vi "motionMagicConfig.vi"() -> ()   [LabVIEW 2018]
uses:
  conversionTypeEnum.ctl
  Constants.vi
panel:
  out "Max Velocity (Inches)":dbl=3.9081455805892547
  in  "D":dbl
  in  "I":dbl
  in  "P":dbl=3.0
  in  "Acceleration":i32=6000
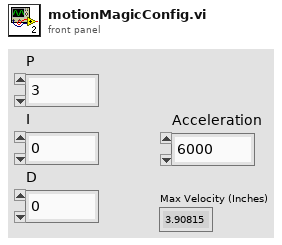
[diagram p1: front panel]
types:
  T1 = typedef "conversionTypeEnum.ctl" = enum16{"Sensor Units -> Inches", "Inches -> Sensor Units"}
  T2 = typedef "WPI_MotorControlDeviceRef.ctl" = cluster{"DeviceStatus":errorcluster, "Type":T3, "PWM":cluster{"PWM Channel":T4, "DeadBand":T5}, "CAN":cluster{"Device Number":u8, "SetOutput VI Ref":variant, "GetOutput VI Ref":variant, "Enable VI Ref":variant, "Disable VI Ref":variant, "Data":variant}, "Invert":bool, "DIO PWM":cluster{"PWM \"Enable\" Channel":T4, "DIOChannel":T6, "PWM Rate":dbl}}
  T3 = typedef "WPI_MotorControlType.ctl" = enum16{"PWM", "CAN", "DIO PWM"}
  T4 = typedef "FPGA_DIOPWMChannel.ctl" = enum8{"PWM 0", "PWM 1", "PWM 2", "PWM 3", "PWM 4", "PWM 5", "PWM 6", "PWM 7", "PWM 8", "PWM 9", "PWM MXP 0", "PWM MXP 1", "PWM MXP 2", "PWM MXP 3", "PWM MXP 4", "PWM MXP 5", "PWM MXP 6", "PWM MXP 7", "PWM MXP 8", "PWM MXP 9", "Invalid"}
  T5 = typedef "WPI_PWMDeadband.ctl" = cluster{"Name":string, "maxPositivePwm":i32, "minPositivePwm":i32, "centerPwm":i32, "maxNegativePwm":i32, "minNegativePwm":i32, "angularRange":u16}
  T6 = typedef "FPGA_DIOChannel.ctl" = enum8{"DIO 0", "DIO 1", "DIO 2", "DIO 3", "DIO 4", "DIO 5", "DIO 6", "DIO 7", "DIO 8", "DIO 9", "DIO MXP 0", "DIO MXP 1", "DIO MXP 2", "DIO MXP 3", "DIO MXP 4", "DIO MXP 5", "DIO MXP 6", "DIO MXP 7", "DIO MXP 8", "DIO MXP 9", "DIO MXP 10", "DIO MXP 11", "DIO MXP 12", "DIO MXP 13", "DIO MXP 14", "DIO MXP 15", "SPI Port CS1", "SPI Port CS2", "SPI Port CS3", "SPI Port MISO", "SPI Port MOSI", "Invalid"}
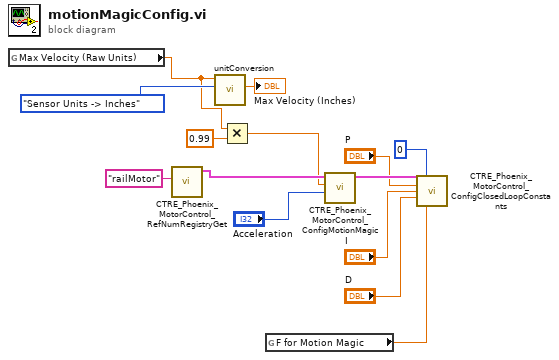
[diagram p0: block diagram]
diagram:
  n1 = global read "Constants.vi" "Max Velocity (Raw Units)"() -> (w3:dbl)
  n2 = call <vilib>:"CTRE_Phoenix_MotorControl_RefNumRegistryGet.vi"("refnum name"="railMotor") -> ("PhoenixMotorControlDevRef"=w13:T2)  [unwired: 9 in, 1 out]
  n3 = call "unitConversion.vi"("Conversion Type"=conversionTypeEnum."Sensor Units -> Inches", "Units to Convert"=w3) -> ("Conversion Result"=→"Max Velocity (Inches)":dbl)  [unwired: 9 in]
  n4 = Multiply(x=w3, y=0.99) -> (x*y=w1:dbl)
  n5 = global read "Constants.vi" "F for Motion Magic"() -> (w6:dbl)
  n6 = call <vilib>:"CTRE_Phoenix_MotorControl_ConfigMotionMagic.vi"("Acceleration"="Acceleration", "Cruise Velocity"=w1, "PhoenixMotorControlDevRef"=w13) -> ("PhoenixMotorControlDevRef"=w11:T2)  [unwired: 7 in, 1 out]
  n7 = call <vilib>:"CTRE_Phoenix_MotorControl_ConfigClosedLoopConstants.vi"("PhoenixMotorControlDevRef"=w11, "slotIdx"=0, "P"="P", "I"="I", "D"="D", "F"=w6) -> ()  [unwired: 8 in, 2 out]
